vi "Event Select User.vi"(8 "error in (no error)":errorcluster, 11 "[V] Login in":refnum<class "[V] Login.lvclass">) -> (0 "error out":errorcluster, 3 "[V] Login out":refnum<class "[V] Login.lvclass">)   [LabVIEW 2020, in "[V] Login.lvlib" / "[V] Login.lvclass"]
uses:
  [V] Login.lvclass
  [V] Login.lvclass/[V] Login.ctl
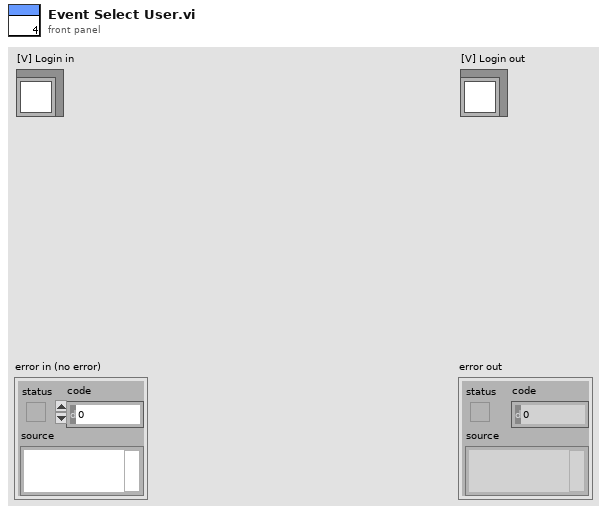
[diagram p1: front panel]
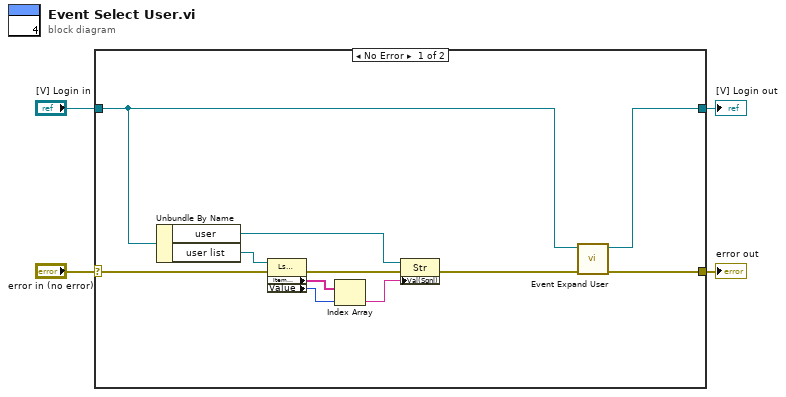
[diagram p0: block diagram]
diagram:
  n1 = case shown="No Error" "error in (no error)" {
    selector: "error in (no error)" -> [w12 w17]
    tunnel: [w15 w17] -> w3
    tunnel: [w14 w16] -> w1
    tunnel: "[V] Login in" -> [w13 w16]
    frame No Error {
      n2 = Unbundle By Name(w13) -> ("user"=w7:refnum<vi>, "user list"=w11:refnum<vi>)
      n3 = property class="LstBox (strict)"(reference=w11, error in=w12) -> (error out=w8:errorcluster, "Item Names"=w10:string[], "Value"=w9:i32)  [unwired: 1 out]
      n4 = Index Array(array=w10, index=w9) -> (element=w6:string)
      n5 = property class="Str"(reference=w7, error in=w8, "Val(Sgnl)"=w6) -> (error out=w5:errorcluster)  [unwired: 1 out]
      n6 = call "Event Expand User.vi"("error in (no error)"=w5, "[V] Login in"=w13) -> ("error out"=w15:errorcluster, "[V] Login out"=w14:refnum<class "[V] Login.lvclass">)  [unwired: 8 in]
    }
    frame Error {
    }
  }
  "error out" <- w3
  "[V] Login out" <- w1
